vi "vCE_ExeVersionInformation.vi"(8 "error in (no error)":errorcluster) -> (0 "error out":errorcluster, 3 "FileVersion":string)   [LabVIEW 2014, in "FPGADMAChannelData.lvclass"]
uses:
  FPGADMAChannelData.lvclass
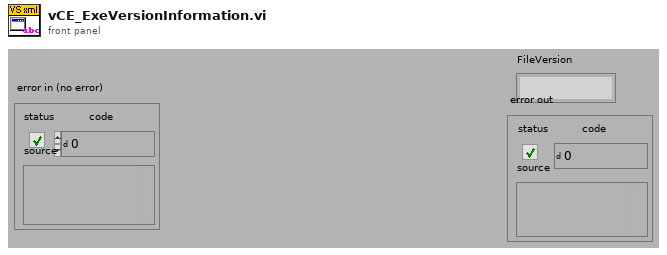
[diagram p1: front panel]
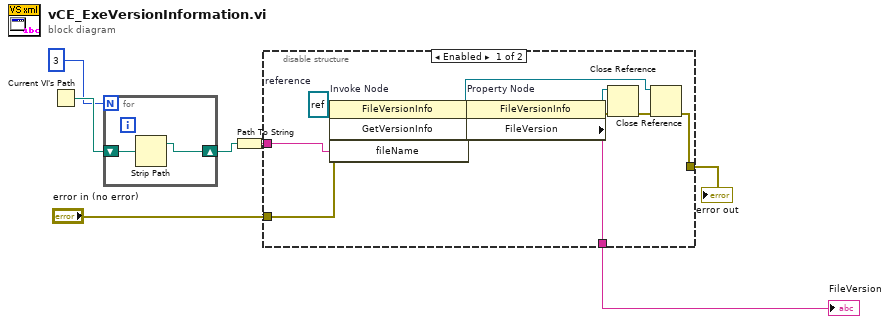
[diagram p0: block diagram]
diagram:
  n1 = Current VI's Path() -> (path=w7:path)
  n2 = for {
    N: 3 -> [_]
    shift-right: [w8] -> w6
    shift-left: w7 -> [w9]
    n3 = Strip Path(path=w9) -> (stripped path=w8:path)  [unwired: 1 out]
  }
  n4 = Path To String(path=w6) -> (string=w5:string)
  n5 = disable-structure shown="Enabled" {
    disable-tunnel: w5 -> [w19 w22]
    disable-tunnel: [w16 w22] -> w4
    disable-tunnel: "error in (no error)" -> [w11 w21]
    disable-tunnel: [w10 w21] -> w2
    frame Enabled {
      w20 = refnum<k24> refnum  # reference
      n6 = invoke on="Invoke Node" class="FileVersionInfo" method="GetVersionInfo"(reference=w20, error in=w11, "fileName"=w19) -> (reference out=w12:refnum<k24>, error out=w17:errorcluster, "GetVersionInfo"=w18:refnum<k24>)  [unwired: 1 in, 1 out]
      n7 = property on="Property Node" class="FileVersionInfo"(reference=w18, error in=w17) -> (reference out=w15:refnum<k24>, error out=w14:errorcluster, "FileVersion"=w16:string)
      n8 = Close Reference(reference=w15, error in (no error)=w14) -> (error out=w13:errorcluster)
      n9 = Close Reference(reference=w12, error in (no error)=w13) -> (error out=w10:errorcluster)
    }
    frame Disabled {
    }
  }
  "FileVersion" <- w4
  "error out" <- w2
